vi "write.vi"() -> ()   [LabVIEW 2020]
panel:
  out "alarma":bool
  in  "stop":bool
  out "Waveform Chart":dynamicdata(graph)
  in  "Temp":dbl(slide) scale=0.0..100.0
  in  "lim 2":dbl
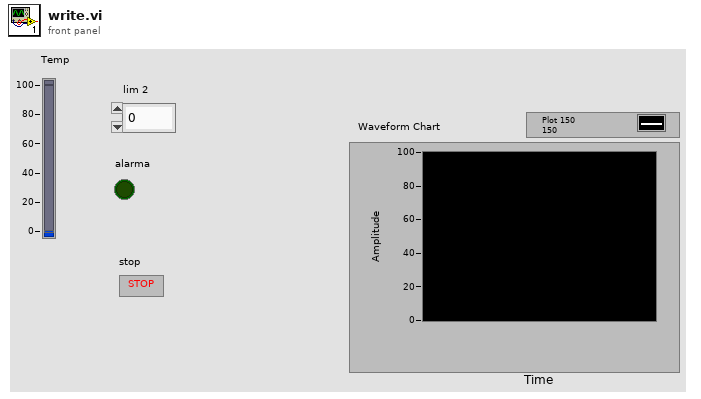
[diagram p1: front panel]
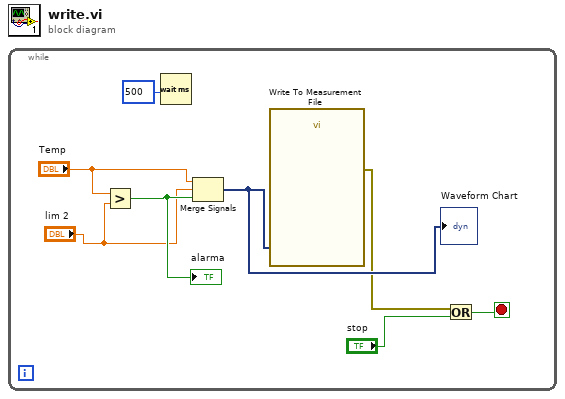
[diagram p0: block diagram]
diagram:
  n1 = while {
    stop <- w7 stop-if-true
    n2 = Greater?(x="Temp", y="lim 2") -> (0:w3:bool)
    "alarma" <- w3
    n3 = Wait (ms)(milliseconds to wait=500) -> ()  [unwired: 1 out]
    n4 = Merge Signals("Temp", "lim 2", w3) -> (w5:dynamicdata)
    "Waveform Chart" <- w5
    n5 = call "Write To Measurement File"("Signals"=w5) -> ("error out"=w4:errorcluster)  [unwired: 16 in, 2 out]
    n6 = Or(x=w4, y="stop") -> (x .or. y?=w7:bool)
  }
